vi "HandleMsg.vi"(0 "reference in":refnum<class "Proccess.lvclass">, 5 "message in":T1, 7 "Unhandled in":bool, 11 "error in (no error)":errorcluster) -> (4 "reference out":refnum<class "Proccess.lvclass">, 6 "message out":T1, 8 "Unhandled out":bool, 15 "error out":errorcluster)   [LabVIEW 2019, in "Proccess.lvclass"]
uses:
  Proccess.lvclass
  MessageInterface_class/Message.ctl
  MessageInterface_class/MessageInterface.lvclass
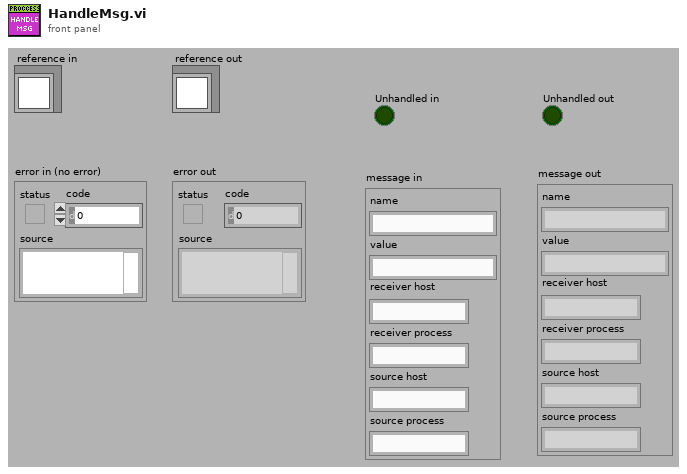
[diagram p1: front panel]
types:
  T1 = typedef "MessageInterface.lvclass/Message.ctl" = cluster{"name":string, "value":string, "receiver host":string, "receiver process":string, "source host":string, "source process":string}
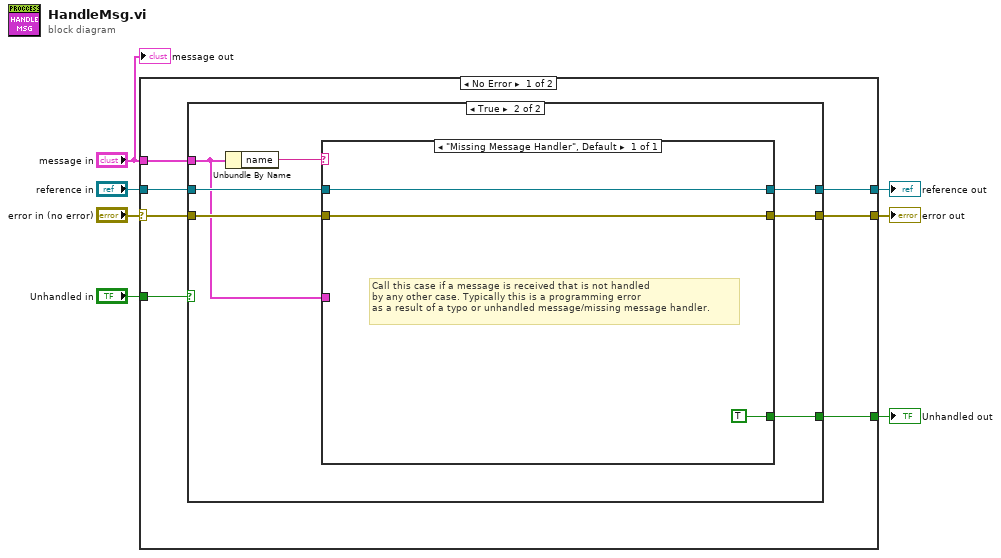
[diagram p0: block diagram]
diagram:
  n1 = case shown="No Error" "error in (no error)" {
    selector: "error in (no error)" -> [w13 w28]
    tunnel: [w10 w28] -> w6
    tunnel: [w12 w27] -> w4
    tunnel: "reference in" -> [w14 w27]
    tunnel: "message in" -> [w11 _]
    tunnel: [w9 _] -> w2
    tunnel: "Unhandled in" -> [w8 _]
    frame No Error {
      n2 = case shown="True" w8 {
        tunnel: w14 -> [w16 w23]
        tunnel: w13 -> [w15 w22]
        tunnel: [w16 w21] -> w12
        tunnel: w11 -> [_ w17]
        tunnel: [w15 w19] -> w10
        tunnel: [_ w18] -> w9
        frame False {
        }
        frame True {
          n3 = Unbundle By Name(w17) -> ("name"=w20:string)
          n4 = case shown="\"Missing Message Handler\", Default" w20 {
            tunnel: [TRUE] -> w18
            tunnel: [w25] -> w21
            tunnel: w23 -> [w25]
            tunnel: [w24] -> w19
            tunnel: w22 -> [w24]
            tunnel: w17 -> [_]
            frame "Missing Message Handler", Default {
              # "Call this case if a message is received that is not handled \nby any other case. Typically this is a programming error\nas a result of a typo or unhandled message/missing message handler."
            }
          }
        }
      }
    }
    frame Error {
    }
  }
  "error out" <- w6
  "reference out" <- w4
  "Unhandled out" <- w2
  "message out" <- "message in"
